vi "Force Extrema Set.vi"(8 "error in (no error)":errorcluster, 9 "Minimum Force (N)":T1={"Fx (N)"=-3.0, "Fy (N)"=-3.0, "Fz (N)"=-3.0} {"Fx (N)" format="%.1f"; "Fy (N)" format="%.1f"; "Fz (N)" format="%.1f"}, 10 "Maximum Force (N)":T1={"Fx (N)"=3.0, "Fy (N)"=3.0, "Fz (N)"=3.0} {"Fx (N)" format="%.1f"; "Fy (N)" format="%.1f"; "Fz (N)" format="%.1f"}) -> (0 "error out":errorcluster)   [LabVIEW 2023, in "Haptic Prog Interface.lvlib"]
doc: "Sets the maximum positive and negative forces the pen can apply.\n\n<b>Maximum Force:</b> A cluster of the maximum positive x, y, and z forces on the pen (in units of N).\n\n<b>Minimum Force:</b> A cluster of the maximum negative x, y, and z forces on the pen (in units of N)."
uses:
  Haptic Prog Interface.lvlib
  Haptic-Programming-Interface/src/x64/Debug/Haptic Programming Interface.dll
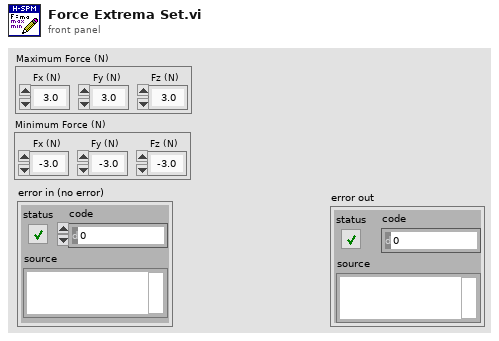
[diagram p1: front panel]
types:
  T1 = cluster{"Fx (N)":dbl, "Fy (N)":dbl, "Fz (N)":dbl}
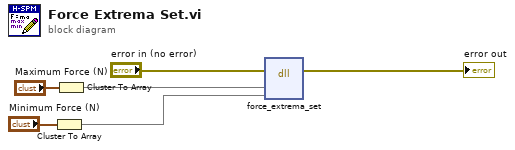
[diagram p0: block diagram]
diagram:
  n1 = Cluster To Array(cluster="Minimum Force (N)") -> (array=w1:dbl[])
  n2 = Cluster To Array(cluster="Maximum Force (N)") -> (array=w3:dbl[])
  n3 = dll-call lib="C:/Users/cjwel/Documents/GitHub/Haptic-Programming-Interface/src/x64/Debug/Haptic Programming Interface.dll" fn="force_extrema_set"(error in="error in (no error)", "maxforce"=w3, "minforce"=w1) -> (error out=→"error out":errorcluster)  [unwired: 5 in, 1 out]
